vi "write keyword - float.vi"(8 "error in (no error)":errorcluster, 9 "Value":dbl, 10 "keyword":string, 11 "Simulated_Header in":refnum<class "Simulated_Header.lvclass">) -> (0 "error out":errorcluster, 3 "Simulated_Header out":refnum<class "Simulated_Header.lvclass">)   [LabVIEW 2018, in "Simulated_Header.lvclass"]
uses:
  Simulated_Header.lvclass
  Simulated_Header.lvclass/Simulated_Header.ctl
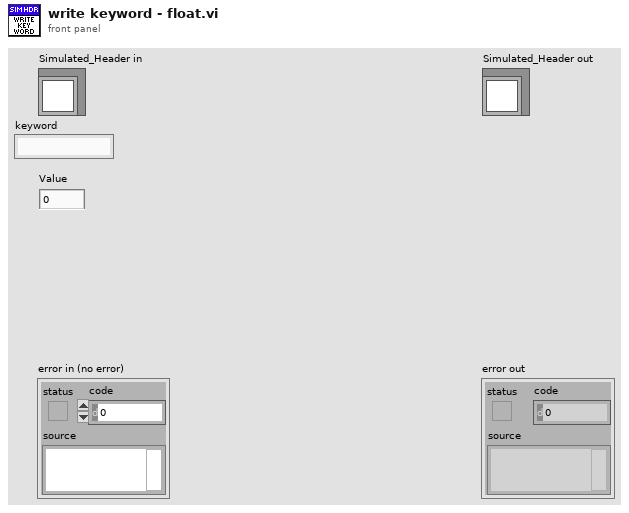
[diagram p1: front panel]
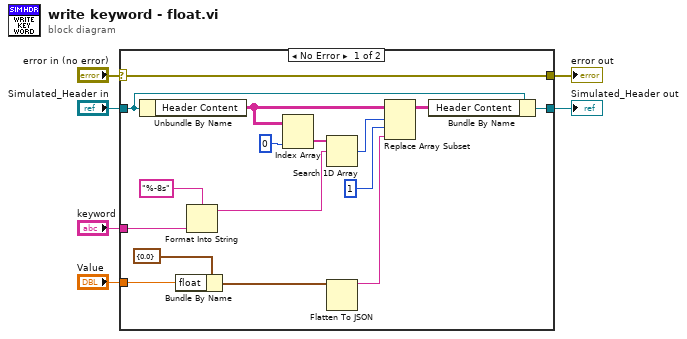
[diagram p0: block diagram]
diagram:
  n1 = case shown="No Error" "error in (no error)" {
    selector: "error in (no error)" -> [w22 w24]
    tunnel: [w22 w24] -> w5
    tunnel: [w15 w23] -> w3
    tunnel: "Simulated_Header in" -> [w16 w23]
    tunnel: "keyword" -> [w8 _]
    tunnel: "Value" -> [w13 _]
    frame No Error {
      n2 = Unbundle By Name(w16) -> ("Header Content"=w19:string[][])
      n3 = Bundle By Name(cluster=cluster{"float":dbl} {"float"=0.0}, "float"=w13) -> (w12:cluster{"float":dbl})
      n4 = Format Into String(format string="%-8s", w8) -> (resulting string=w7:string)  [unwired: 2 in, 1 out]
      n5 = Index Array(array=w19, index (col)=0 ("disabled index (col)")) -> (element=w20:string[])  [unwired: 1 in]
      n6 = Search 1D Array(1D array=w20, element=w7) -> (index of element=w17:i32)  [unwired: 1 in]
      n7 = Flatten To JSON(anything=w12) -> (JSON string=w11:string)  [unwired: 2 in, 1 out]
      n8 = Replace Array Subset(array=w19, new element=w11, index (row)=w17, index (col)=1 ("disabled index (col)")) -> (w10:string[][])
      n9 = Bundle By Name(cluster=w16, "Header Content"=w10) -> (w15:refnum<class "Simulated_Header.lvclass">)
    }
    frame Error {
    }
  }
  "error out" <- w5
  "Simulated_Header out" <- w3
